vi "Get Temperature Range.vi"(10 "maxtemp":i32, 11 "mintemp":i32) -> (1 "function return":u32, 2 "maxtemp out":i32, 3 "mintemp out":i32)   [LabVIEW 2018, in "Copy of Andor SDK.lvlib"]
doc: "EXPNETTYPE unsigned int WINAPI GetTemperatureRange(int * mintemp, int * maxtemp);"
uses:
  Copy of Andor SDK.lvlib
  <userlib>/Andor SDK/ATMCD32D.dll
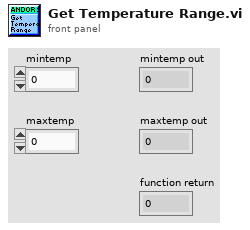
[diagram p1: front panel]
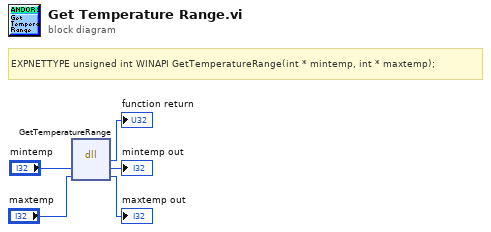
[diagram p0: block diagram]
diagram:
  # "EXPNETTYPE unsigned int WINAPI GetTemperatureRange(int * mintemp, int * maxtemp);"
  n1 = dll-call lib="C:/Program Files (x86)/National Instruments/LabVIEW 2018/user.lib/Andor SDK/ATMCD32D.*" fn="GetTemperatureRange"("mintemp"="mintemp", "maxtemp"="maxtemp") -> (→"function return":u32, "mintemp"=→"mintemp out":i32, "maxtemp"=→"maxtemp out":i32)  [unwired: 3 in, 2 out]
